vi "Stop Core.vi"(10 "final error code":i32, 11 "Actor1_GUI in":refnum<class "Tesla Tester GUI.lvclass">) -> (3 "Actor1_GUI out":refnum<class "Tesla Tester GUI.lvclass">)   [LabVIEW 2013, in "Tesla Tester GUI.lvlib" / "Tesla Tester GUI.lvclass"]
doc: "(<B>Filename</B>: Actor Framework.lvlib:Actor.lvclass:Stop Core.vi)\n\nDefines what the actor does before it stops. Use the <B>final error code</B> input to determine whether the actor shut down in response to an error.\n\nBy default, this method does nothing. A descendant class may override it to define behavior, such as shutting down any processes the actor initiated in its override of the Actor Core method."
uses:
  Tesla Tester GUI.lvclass
  <vilib>/ActorFramework/Actor/Actor.lvclass
  Tesla Tester GUI.lvclass/Tesla Tester GUI.ctl
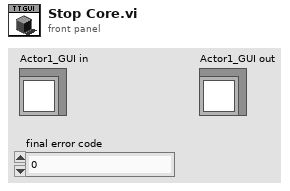
[diagram p1: front panel]
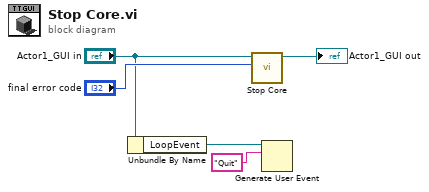
[diagram p0: block diagram]
diagram:
  n1 = Unbundle By Name("Actor1_GUI in") -> ("LoopEvent"=w2:refnum<user-event>)
  n2 = call-parent "Stop Core.vi"("final error code"="final error code", "Actor in"="Actor1_GUI in") -> ("Actor out"=→"Actor1_GUI out":refnum<class "Tesla Tester GUI.lvclass">)  [unwired: 9 in]
  n3 = Generate User Event(user event=w2, event data cluster="Quit" ("event data")) -> ()  [unwired: 2 in, 2 out]
